vi "Read atime and mtime.vi"(8 "error in (no error)":errorcluster, 11 "file attributes in":refnum<class "File Attributes.lvclass">) -> (0 "error out":errorcluster, 2 "atime/mtime":cluster{"atime":u32, "mtime":u32}, 3 "file attributes out":refnum<class "File Attributes.lvclass">)   [LabVIEW 2020, in "NI_SFTP.lvlib" / "File Attributes.lvclass"]
doc: "Reads the access and modification time stored in this File Attributes object, returning Unix timestamps.\n\nThis property may not always be populated by SFTP VIs. If it does not exist, an error is returned."
uses:
  <vilib>/net/SFTP/File Attributes/File Attributes.lvclass
  <vilib>/net/SFTP/File Attributes/File Attributes.lvclass/File Attributes.ctl
  <vilib>/Utility/error.llb/Error Cluster From Error Code.vi
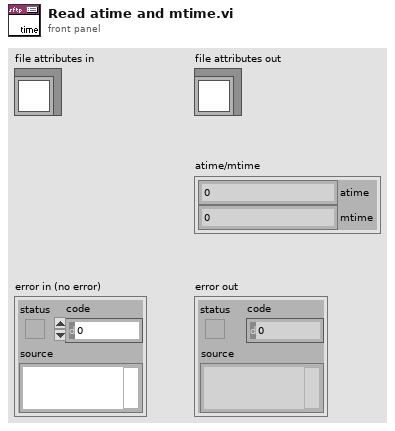
[diagram p1: front panel]
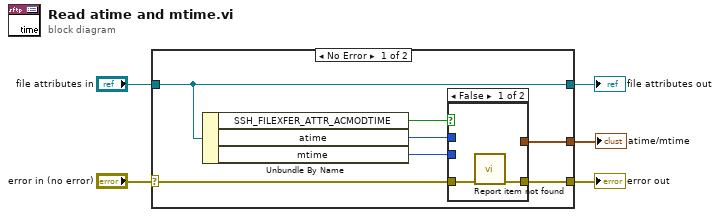
[diagram p0: block diagram]
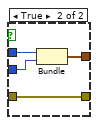
[diagram p2: hidden frame]
diagram:
  n1 = case shown="No Error" "error in (no error)" {
    selector: "error in (no error)" -> [w7 w19]
    tunnel: [w8 w19] -> w4
    tunnel: [w12 w20] -> w2
    tunnel: "file attributes in" -> [w12 w20]
    tunnel: [w9 _] -> w1
    frame No Error {
      n2 = Unbundle By Name(w12) -> ("SSH_FILEXFER_ATTR_ACMODTIME"=w6:bool, "atime"=w11:u32, "mtime"=w10:u32)
      n3 = case shown="False" w6 {
        tunnel: w11 -> [_ w18]
        tunnel: w10 -> [_ w17]
        tunnel: [_ w16] -> w9
        tunnel: [w13 w15] -> w8
        tunnel: w7 -> [w14 w15]
        frame False {
          n4 = call <vilib>:"Report item not found.vi"("error in (no error)"=w14) -> ("error out"=w13:errorcluster)  [unwired: 10 in]
        }
        frame True {
          n5 = Bundle("atime"=w18, "mtime"=w17) -> (w16:cluster{"atime":u32, "mtime":u32})  [unwired: 1 in]
        }
      }
    }
    frame Error {
    }
  }
  "error out" <- w4
  "file attributes out" <- w2
  "atime/mtime" <- w1
